vi "Waterfall Plot.vi"() -> ()   [LabVIEW 2014]
doc: "This example uses the CW3Dgraph ActiveX Object to create a Waterfall plot using. The VI uses Express VIs to generate a sine wave and calculate the FFT Power spectrum. The result is plotted in a 3D graph using a feedback node to build the Z-Matrix. A shift register is used to build the Z-Matrix."
uses:
  <vilib>/addons/_XControls/Waterfall Graph/SVX Waterfall Graph.xctl
  <vilib>/express/express analysis/Spectral/Block/exnSpectralBlock spectral measurements power poly.vi
  <vilib>/express/express analysis/Spectral/Block/exnSpectralBlock spectral measurements power WFM.vi
  <vilib>/addons/_XControls/Utility/SVX Buffer Waterfall Graph (Single Plot).vi
  <vilib>/express/express analysis/Spectral/XNode/ExpressSpectralMeasurementsBlockNode.xnode
  <vilib>/addons/Sound and Vibration/Order Analysis/Data Presentation/SoundVib_SpectralDisplay.lvlib
panel:
  out "Sine Wave with noise":dynamicdata(graph)
  in  "Amplitude":dbl(knob)=3.0308604113585513 scale=0.0..6.0 scale format="%#_2g"
  in  "Frequency":dbl(knob)=50.9891320903669 scale=0.0..500.0
  out "Waterfall Graph":T1(xcontrol)={"z0"=0.0, "dz"=1.0, "Plots"=[]}
  in  "stop":bool
  # "You can tilt the aspect of the graph by holding Ctrl and dragging with the mouse"
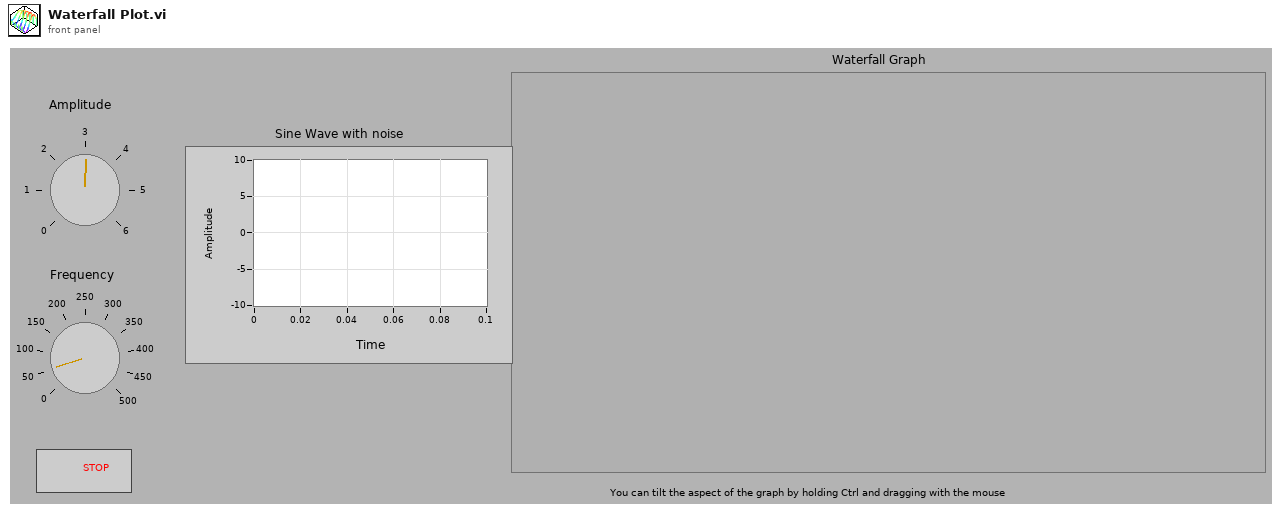
[diagram p1: front panel]
types:
  T1 = cluster{"z0":dbl, "dz":dbl, "Plots":cluster{"x0":dbl, "dx":dbl, "Y":dbl[]}[]}
  T2 = cluster{"averaging mode":u16, "weighting mode":u16, "number of averages":u32}
  T3 = cluster{"dB On (F)":bool, "unwrap phase (F)":bool, "convert to degree (F)":bool}
  T4 = cluster{"z0":dbl, "dz":dbl, "plots":cluster{"x0":dbl, "dx":dbl, "Y":dbl[]}[]}
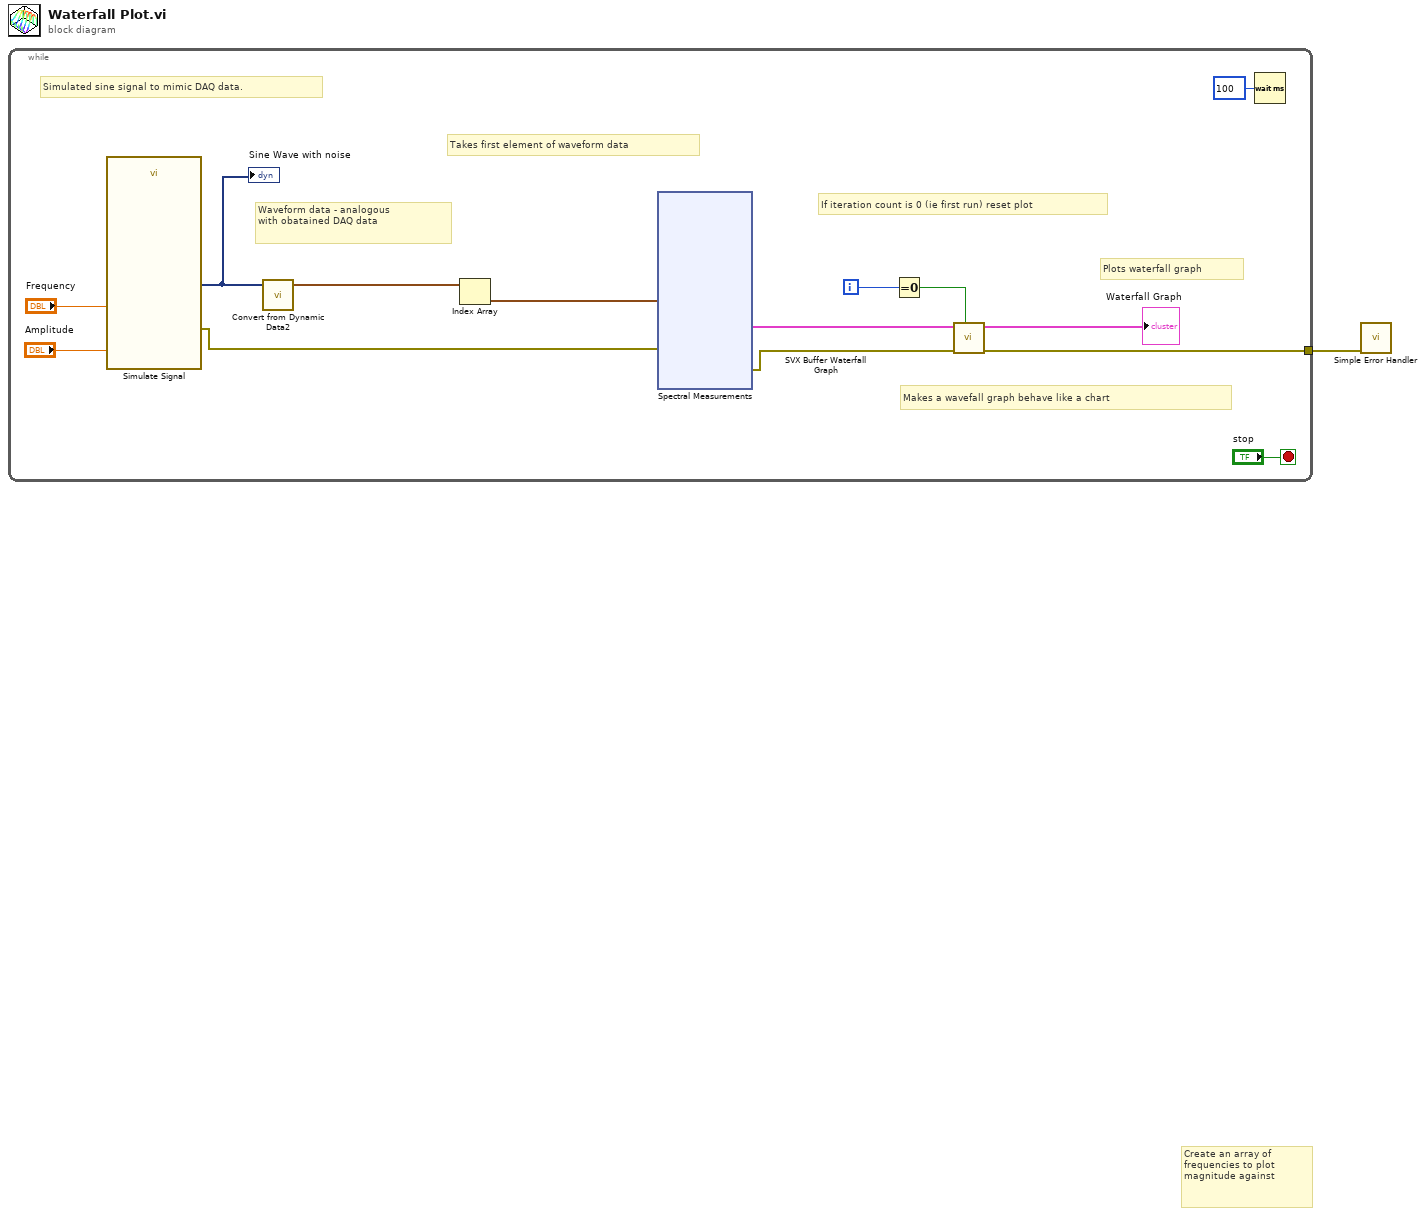
[diagram p0: block diagram]
diagram:
  # "Create an array of \nfrequencies to plot\nmagnitude against"
  n1 = while {
    tunnel: [w9] -> w1
    i -> [w2]
    stop <- "stop" stop-if-true
    # "Plots waterfall graph"
    # "Makes a wavefall graph behave like a chart"
    # "If iteration count is 0 (ie first run) reset plot"
    # "Takes first element of waveform data"
    # "Waveform data - analogous \nwith obatained DAQ data"
    # "Simulated sine signal to mimic DAQ data."
    n2 = call "Simulate Signal"("Frequency"="Frequency", "Amplitude"="Amplitude") -> ("Sine with Gaussian Noise"=w3:dynamicdata, "error out"=w7:errorcluster)  [unwired: 12 in]
    "Sine Wave with noise" <- w3
    n3 = call "Convert from Dynamic Data2"("Dynamic Data Type"=w3) -> ("Array of Waveform"=w14:waveform(dbl)[])  [unwired: 3 in]
    n4 = Index Array(array=w14) -> (element=w13:waveform(dbl))  [unwired: 1 in]
    n5 = xnode "Spectral Measurements"("Signals"=w13, "error in (no error)"=w7) -> ("Power Spectrum"=w4:cluster{"f0":dbl, "df":dbl, "magnitude":dbl[]}, "error out"=w8:errorcluster)
    n6 = Equal To 0?(x=w2) -> (x = 0?=w10:bool)
    n7 = call-poly <vilib>:"SVX Buffer Waterfall Graph.vi"("reset? (F)"=w10, "error in (no error)"=w8, "plot"=w4) -> ("error out"=w9:errorcluster, "waterfall graph data out"=→"Waterfall Graph":T4)  [unwired: 7 in]
    n8 = Wait (ms)(milliseconds to wait=u32 100) -> ()  [unwired: 1 out]
  }
  n9 = call <vilib>:"Simple Error Handler.vi"("error in (no error)"=w1) -> ()  [unwired: 4 in, 5 out]
